vi "About.vi"() -> ()   [LabVIEW 2011]
panel:
  out "error out":errorcluster
  in  "error in (no error)":errorcluster
  # "File Archive & FTP \nVersion 4.0 Beta\n\nUSGS\nColumbia River Research Laboritory\n5501-A Cookunderwood Rd.\nCook, WA 98605\n(509) 538-2299\n\n\n\n\n\n\n\n\n\n\nDeveloped by: USGS_CRRL_3D\nNovember 8, 2012\nDevelopment platform:\nLabview 2011"
  # "NODE Archive\n&\nFTP File Handler"
  # "ABOUT Diolog"
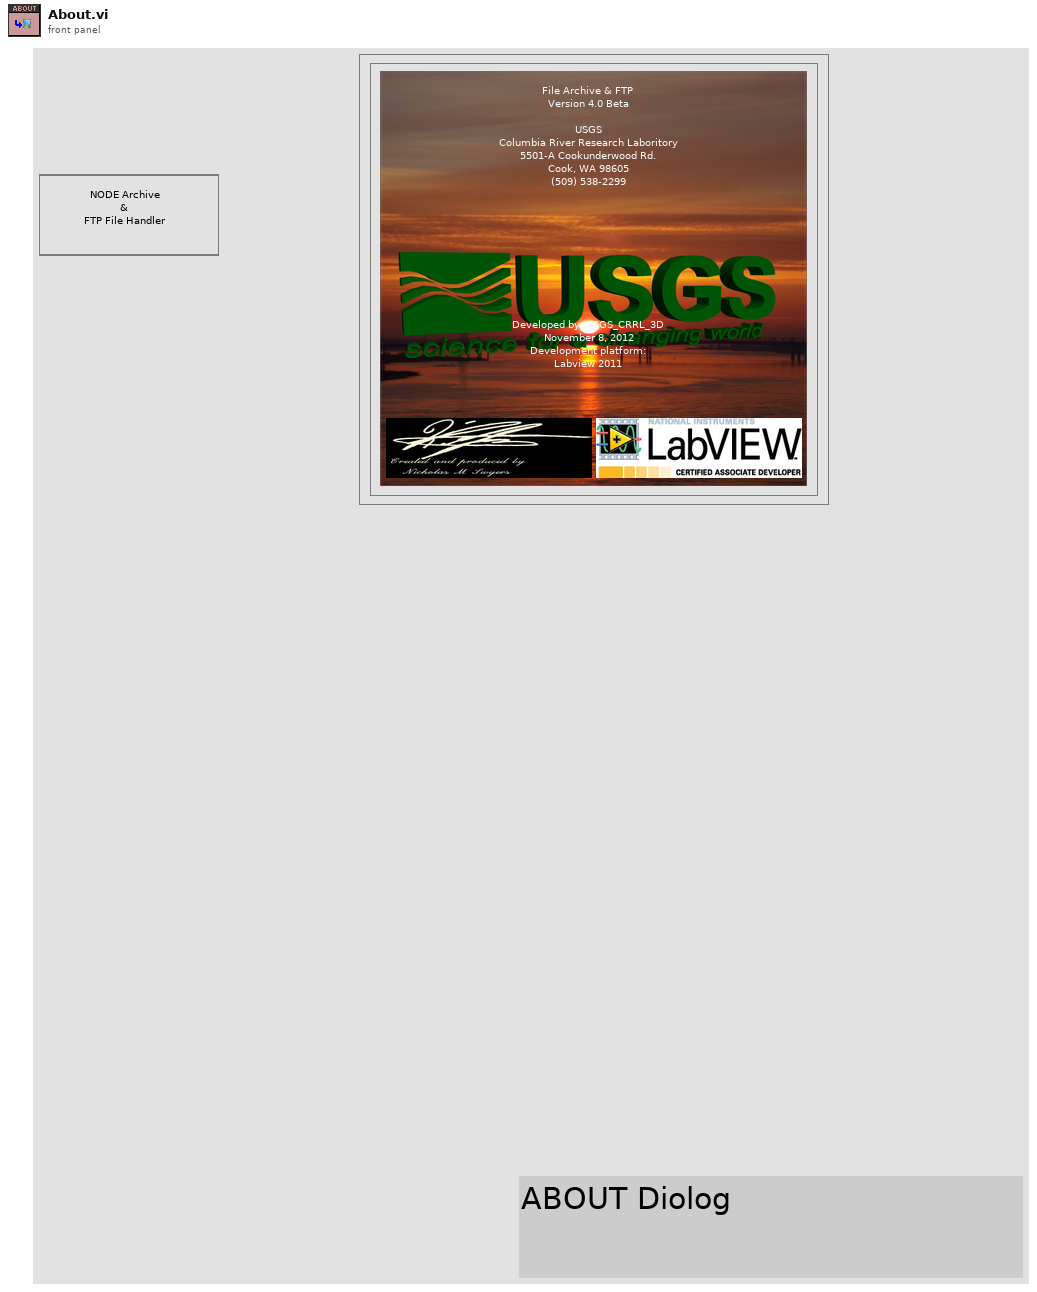
[diagram p1: front panel]
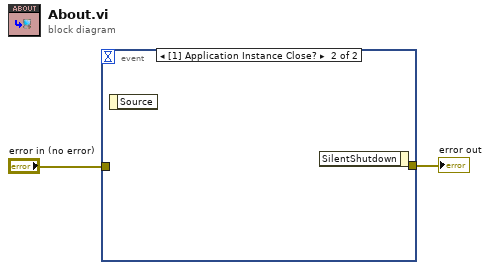
[diagram p0: block diagram]
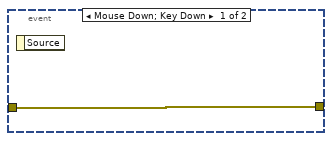
[diagram p2: hidden frame]
diagram:
  n1 = event shown="[1] Application Instance Close?" {
    selector: _ -> [_ _]
    dyn-events: _ -> [_ _]
    timeout: _ -> [_ _]
    tunnel: [w3 _] -> w2
    tunnel: "error in (no error)" -> [w3 _]
    event Mouse Down; Key Down {
      n2 = event-data() -> ()  [unwired: 1 in, 1 out]
    }
    event Application Instance Close? {
      n3 = event-data() -> ()  [unwired: 1 in, 1 out]
      n4 = event-data() -> ()  [unwired: 2 in, 1 out]
    }
  }
  "error out" <- w2
